vi "Generator.vi"(6 "Sampling Info":cluster{"Fs":dbl, "#s":dbl}, 8 "error in (no error)":errorcluster, 10 "Messenger Type (Sine)":enum16{"Sine", "Sawtooth", "Square", "Triangle"}(ring), 11 "Messenger Control":T1={"Frequency (Hz)"=10.0, "Amplitude (V)"=1.0, "Phase (°)"=0.0}) -> (0 "error out":errorcluster, 3 "Signal Out":waveform(dbl))   [LabVIEW 2020]
uses:
  <vilib>/measure/NI_MABase.lvlib
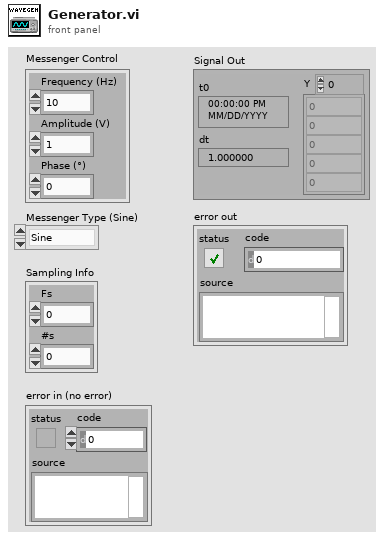
[diagram p1: front panel]
types:
  T1 = cluster{"Frequency (Hz)":dbl, "Amplitude (V)":dbl, "Phase (°)":dbl}
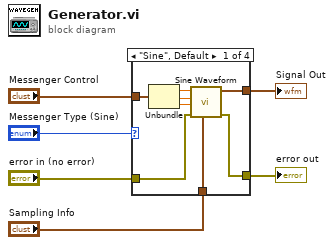
[diagram p0: block diagram]
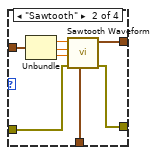
[diagram p2: hidden frame]
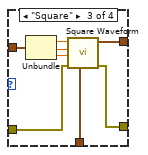
[diagram p3: hidden frame]
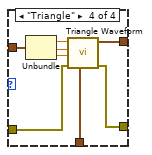
[diagram p4: hidden frame]
diagram:
  n1 = case shown="\"Sine\", Default" "Messenger Type (Sine)" {
    tunnel: "Messenger Control" -> [w14 w22 w30 w38]
    tunnel: [w10 w18 w26 w34] -> w5
    tunnel: "Sampling Info" -> [w9 w17 w25 w33]
    tunnel: "error in (no error)" -> [w7 w16 w23 w32]
    tunnel: [w8 w15 w24 w31] -> w2
    frame "Sine", Default {
      n2 = Unbundle(w14) -> ("Frequency (Hz)"=w13:dbl, "Amplitude (V)"=w12:dbl, "Phase (°)"=w11:dbl)
      n3 = call <vilib>:"Sine Waveform.vi"("sampling info"=w9, "error in (no error)"=w7, "phase"=w11, "amplitude"=w12, "frequency"=w13) -> ("error out"=w8:errorcluster, "signal out"=w10:waveform(dbl))  [unwired: 5 in]
    }
    frame "Sawtooth" {
      n4 = Unbundle(w22) -> ("Frequency (Hz)"=w21:dbl, "Amplitude (V)"=w20:dbl, "Phase (°)"=w19:dbl)
      n5 = call <vilib>:"Sawtooth Waveform.vi"("sampling info"=w17, "error in (no error)"=w16, "phase"=w19, "amplitude"=w20, "frequency"=w21) -> ("error out"=w15:errorcluster, "signal out"=w18:waveform(dbl))  [unwired: 5 in]
    }
    frame "Square" {
      n6 = Unbundle(w30) -> ("Frequency (Hz)"=w29:dbl, "Amplitude (V)"=w28:dbl, "Phase (°)"=w27:dbl)
      n7 = call <vilib>:"Square Waveform.vi"("sampling info"=w25, "error in (no error)"=w23, "phase"=w27, "amplitude"=w28, "frequency"=w29) -> ("error out"=w24:errorcluster, "signal out"=w26:waveform(dbl))  [unwired: 5 in]
    }
    frame "Triangle" {
      n8 = Unbundle(w38) -> ("Frequency (Hz)"=w37:dbl, "Amplitude (V)"=w36:dbl, "Phase (°)"=w35:dbl)
      n9 = call <vilib>:"Triangle Waveform.vi"("sampling info"=w33, "error in (no error)"=w32, "phase"=w35, "amplitude"=w36, "frequency"=w37) -> ("error out"=w31:errorcluster, "signal out"=w34:waveform(dbl))  [unwired: 5 in]
    }
  }
  "Signal Out" <- w5
  "error out" <- w2
